vi "AcqFromFil.vi"() -> ()   [LabVIEW 2017]
uses:
  <vilib>/sound2/lvsound2.llb/Sound Data Format.ctl
  <vilib>/sound2/lvsound2.llb/Sampling Mode.ctl
  <vilib>/sound2/lvsound2.llb/Sound File Write Open.vi
  <vilib>/sound2/lvsound2.llb/Sound Input Read (DBL).vi
  <vilib>/sound2/lvsound2.llb/Sound File Write (DBL).vi
panel:
  out "Waveform Graph":waveform(dbl)[](graph)
  in  "path":path
  in  "stop":bool
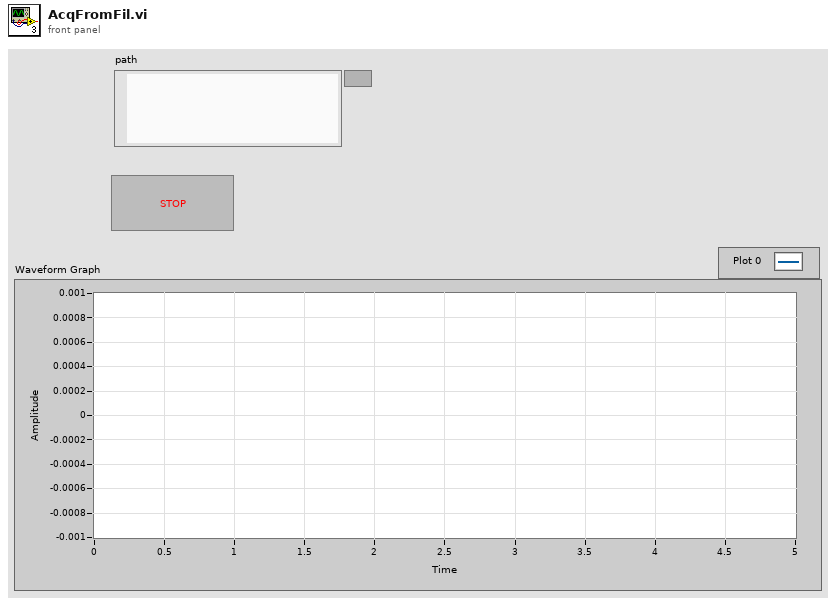
[diagram p1: front panel]
types:
  T1 = typedef "Sampling Mode.ctl" = i32
  T2 = typedef "Sound Data Format.ctl" = cluster{"sample rate (S/s)":dbl, "number of channels":i32, "bits per sample":i32}
  T3 = typedef "Sound File Refnum.ctl" = refnum<file>
  T4 = typedef "Sound Input Task ID.ctl" = u32
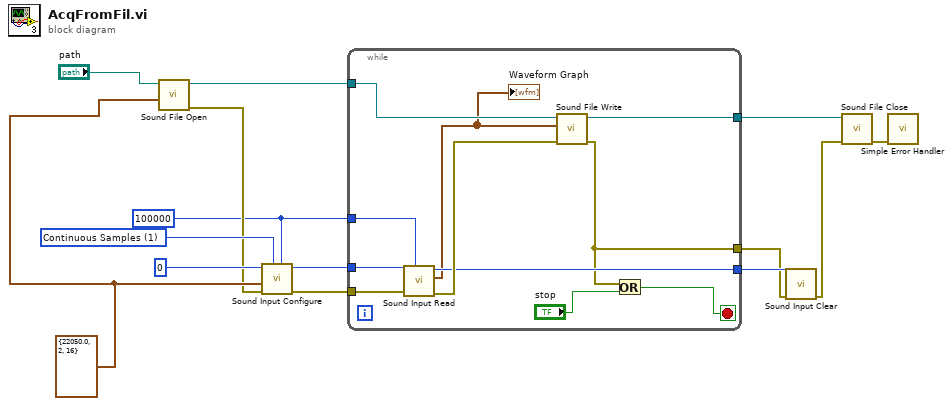
[diagram p0: block diagram]
diagram:
  w8 = 100000 ("number of samples/ch")
  w13 = T1 1 items=["Finite Samples", "Continuous Samples"] ("sample mode")
  w12 = T2 {"sample rate (S/s)"=22050.0, "number of channels"=2, "bits per sample"=16} ("sound format")
  n1 = call-poly <vilib>:"Sound File Open.vi"("sound format"=w12, "path"="path") -> ("error out"=w11:errorcluster, "sound file refnum"=w7:T3)  [unwired: 8 in]
  n2 = call <vilib>:"Sound Input Configure.vi"("number of samples/ch"=w8, "sample mode"=w13, "error in (no error)"=w11, "sound format"=w12, "device ID"=u32 0) -> ("error out"=w9:errorcluster, "task ID"=w10:T4)  [unwired: 5 in]
  n3 = while {
    tunnel: w10 -> [w25]
    tunnel: w9 -> [w24]
    tunnel: w8 -> [w23]
    tunnel: w7 -> [w22]
    tunnel: [w21] -> w5
    tunnel: [w19] -> w6
    tunnel: [w16] -> w3
    stop <- w18 stop-if-true
    n4 = call-poly <vilib>:"Sound Input Read.vi"("number of samples/ch"=w23, "error in (no error)"=w24, "task ID"=w25) -> ("error out"=w20:errorcluster, "data"=w15:waveform(dbl)[], "task ID out"=w19:T4)  [unwired: 6 in]
    "Waveform Graph" <- w15
    n5 = call-poly <vilib>:"Sound File Write.vi"("error in (no error)"=w20, "data"=w15, "sound file refnum"=w22) -> ("error out"=w16:errorcluster, "sound file refnum out"=w21:T3)  [unwired: 7 in]
    n6 = Or(x=w16, y="stop") -> (x .or. y?=w18:bool)
  }
  n7 = call <vilib>:"Sound Input Clear.vi"("error in (no error)"=w3, "task ID"=w6) -> ("error out"=w4:errorcluster)  [unwired: 9 in]
  n8 = call <vilib>:"Sound File Close.vi"("error in (no error)"=w4, "sound file refnum"=w5) -> ("error out"=w2:errorcluster)  [unwired: 9 in]
  n9 = call <vilib>:"Simple Error Handler.vi"("error in (no error)"=w2) -> ()  [unwired: 4 in, 5 out]
